vi "PressureSetup (SubVI).vi"() -> (0 "error out":errorcluster, 3 "Refnum out":refnum<k21>)   [LabVIEW 2016]
uses:
  <vilib>/DAQmx/create/channels.llb/DAQmx Create Channel (AI-Current-Basic).vi
  <resource>/objmgr/daqmx.rc
  <vilib>/DAQmx/configure/timing.llb/DAQmx Timing (Sample Clock).vi
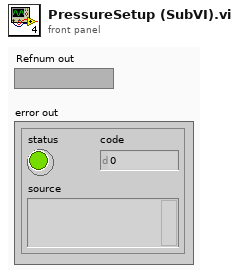
[diagram p1: front panel]
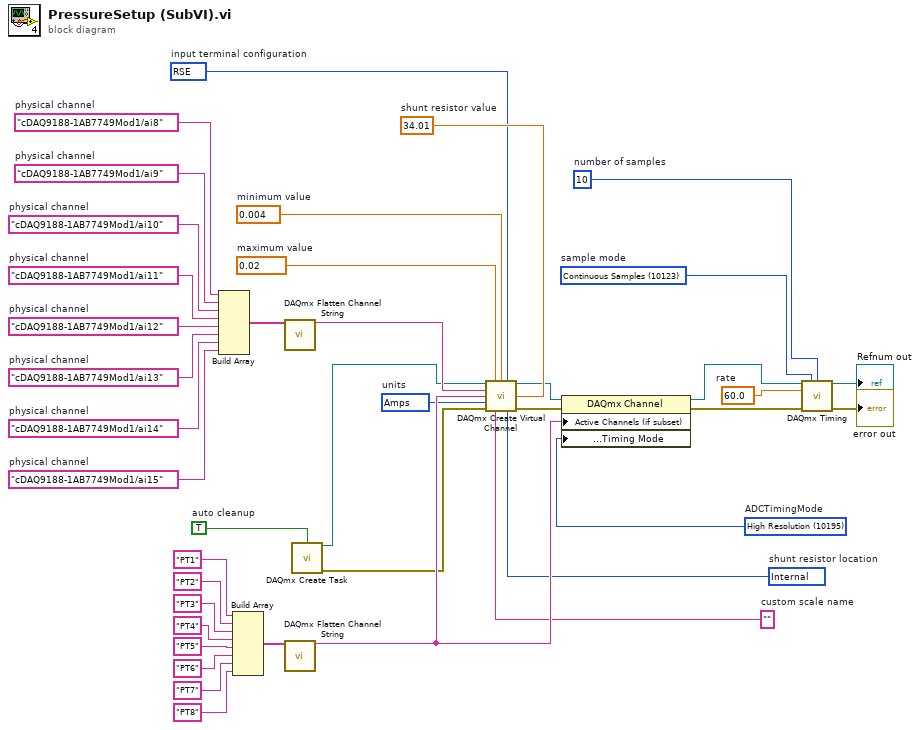
[diagram p0: block diagram]
diagram:
  w35 = "cDAQ9188-1AB7749Mod1/ai11"  # physical channel
  w39 = "cDAQ9188-1AB7749Mod1/ai15"  # physical channel
  w38 = "cDAQ9188-1AB7749Mod1/ai14"  # physical channel
  w37 = "cDAQ9188-1AB7749Mod1/ai13"  # physical channel
  w36 = "cDAQ9188-1AB7749Mod1/ai12"  # physical channel
  w34 = "cDAQ9188-1AB7749Mod1/ai10"  # physical channel
  w33 = "cDAQ9188-1AB7749Mod1/ai9"  # physical channel
  w32 = "cDAQ9188-1AB7749Mod1/ai8"  # physical channel
  w1 = 10123 items=["Finite Samples"=10178, "Continuous Samples"=10123, "Hardware Timed Single Point"=12522]  # sample mode
  w2 = 10  # number of samples
  w3 = 60.0  # rate
  w6 = 10195 items=["High Resolution"=10195, "High Speed"=14712, "Best 50 Hz Rejection"=14713, "Best 60 Hz Rejection"=14714]  # ADCTimingMode
  w8 = 10083 items=["default"=-1, "RSE"=10083, "NRSE"=10078, "Differential"=10106, "Pseudodifferential"=12529]  # input terminal configuration
  w9 = 10342 items=["Amps"=10342, "From Custom Scale"=10065]  # units
  w10 = 34.01  # shunt resistor value
  w11 = 10200 items=["Internal"=10200, "External"=10167]  # shunt resistor location
  w13 = ""  # custom scale name
  w14 = 0.004  # minimum value
  w15 = 0.02  # maximum value
  w17 = TRUE  # auto cleanup
  n1 = Build Array(w32, w33, w34, w35, w36, w37, w38, w39) -> (w40:string[])
  n2 = Build Array("PT1" ("name to assign"), "PT2" ("name to assign"), "PT3" ("name to assign"), "PT4" ("name to assign"), "PT5" ("name to assign"), "PT6" ("name to assign"), "PT7" ("name to assign"), "PT8" ("name to assign")) -> (w22:string[])
  n3 = call <vilib>:"DAQmx Flatten Channel String.vi"("names in"=w40) -> ("names out"=w21:string)  [unwired: 13 in, 1 out]
  n4 = call <vilib>:"DAQmx Flatten Channel String.vi"("names in"=w22) -> ("names out"=w25:string)  [unwired: 13 in, 1 out]
  n5 = call <vilib>:"DAQmx Create Task.vi"("auto cleanup"=w17) -> ("task out"=w16:refnum<k21>, "error out"=w18:errorcluster)  [unwired: 4 in, 9 out]
  n6 = call-poly <vilib>:"DAQmx Create Virtual Channel.vi"("task in"=w16, "maximum value"=w15, "minimum value"=w14, "input terminal configuration"=w8, "physical channels"=w21, "name to assign"=w25, "external shunt resistor value"=w10, "units"=w9, "error in"=w18, "custom scale name"=w13, "shunt resistor location"=w11) -> ("task out"=w5:refnum<k21>, "error out"=w12:errorcluster)  [unwired: 3 out]
  n7 = property class="DAQmx Channel"(reference=w5, error in=w12, "Active Channels (if subset)"=w25, "Analog Input:General Properties:Digitizer/ADC:Timing Mode"=w6) -> (reference out=w4:refnum<k21>, error out=w7:errorcluster)
  n8 = call-poly <vilib>:"DAQmx Timing.vi"("task/channels in"=w4, "sample mode"=w1, "samples per channel"=w2, "rate"=w3, "error in"=w7) -> ("task out"=→"Refnum out":refnum<k21>, "error out"=→"error out":errorcluster)  [unwired: 2 in, 7 out]
